vi "Configure Channel Power.vi"(0 "VISA resource name":refnum<visa-resource-name>, 5 "Channel Power Frequency (3000000000Hz)":dbl=3000000000.0, 7 "Channel Power Bandwidth (31250000Hz)":dbl=31250000.0 min=1.0 max=1000000000.0, 9 "Channel Power Factor (0.22)":dbl=0.22 min=0.01 max=1.0 format="%.2f", 11 "error in (no error)":errorcluster, 12 "Channel Power Filter (0:Rectangular)":i32(ring) items=["Rectangular", "Nyquist", "Root Nyquist"]) -> (4 "VISA resource name out":refnum<visa-resource-name>, 15 "error out":errorcluster)   [LabVIEW 2020, in "Anritsu Signal Analyzer Series.lvlib"]
doc: "Configures the Channel Power settings of the spectrum analyzer."
uses:
  Anritsu Signal Analyzer Series.lvlib
panel:
  # "Hz"
  # "Hz"
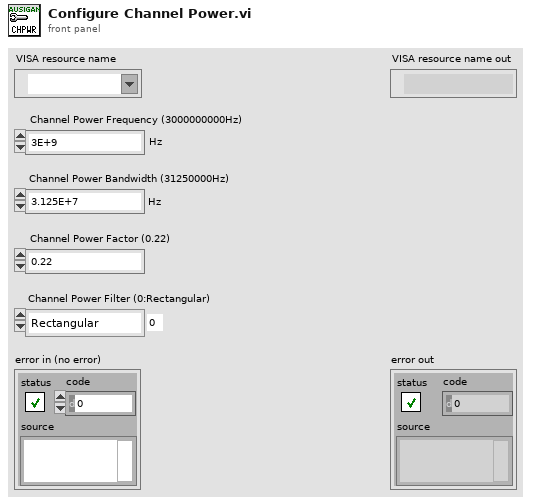
[diagram p1: front panel]
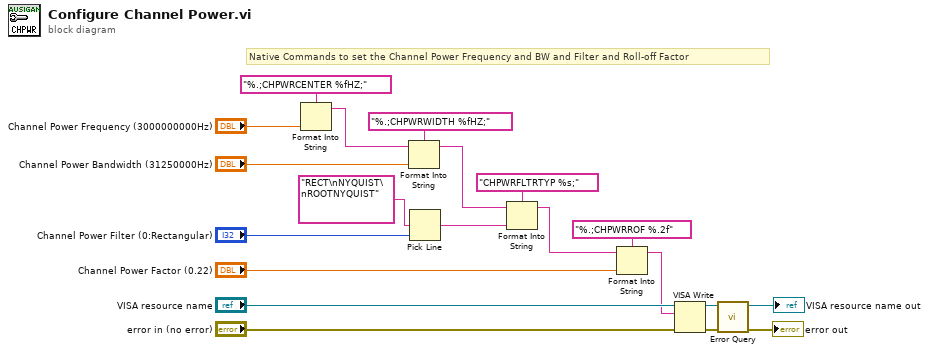
[diagram p0: block diagram]
diagram:
  # "Native Commands to set the Channel Power Frequency and BW and Filter and Roll-off Factor"
  n1 = Format Into String(format string="%.;CHPWRCENTER %fHZ;" ("Format String"), "Channel Power Frequency (3000000000Hz)") -> (resulting string=w10:string)  [unwired: 2 in, 1 out]
  n2 = Format Into String(format string="%.;CHPWRWIDTH %fHZ;" ("Format String"), initial string=w10, "Channel Power Bandwidth (31250000Hz)") -> (resulting string=w8:string)  [unwired: 1 in, 1 out]
  n3 = Pick Line(multi-line string="RECT\nNYQUIST\nROOTNYQUIST" ("複数行文字列"), line index="Channel Power Filter (0:Rectangular)") -> (output string=w1:string)  [unwired: 1 in]
  n4 = Format Into String(format string="CHPWRFLTRTYP %s;" ("_CommandSet"), initial string=w8, w1) -> (resulting string=w6:string)  [unwired: 1 in, 1 out]
  n5 = Format Into String(format string="%.;CHPWRROF %.2f" ("Format String"), initial string=w6, "Channel Power Factor (0.22)") -> (resulting string=w3:string)  [unwired: 1 in, 1 out]
  n6 = VISA Write(VISA resource name="VISA resource name", write buffer=w3, error in (no error)="error in (no error)") -> (VISA resource name out=w5:refnum<visa-resource-name>, error out=w4:errorcluster)  [unwired: 1 out]
  n7 = call "Error Query.vi"("error in (no error)"=w4, "VISA resource name"=w5) -> ("error out"=→"error out":errorcluster, "VISA resource name out"=→"VISA resource name out":refnum<visa-resource-name>)  [unwired: 6 in, 2 out]
